vi "PopulateAscriptTree.vi"(10 "Steps in":T1(array[cluster]), 11 "Autoscript Layout":refnum<vi>) -> (0 "error out":errorcluster, 3 "Autoscript Layout":refnum<vi>)   [LabVIEW 2015]
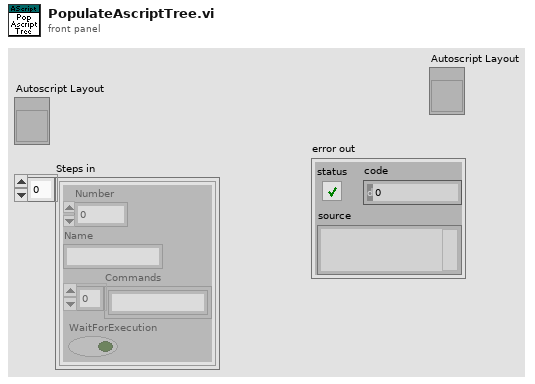
[diagram p1: front panel]
types:
  T1 = cluster{"Number":i32, "Name":string, "Commands":string[], "WaitForExecution":bool}[]
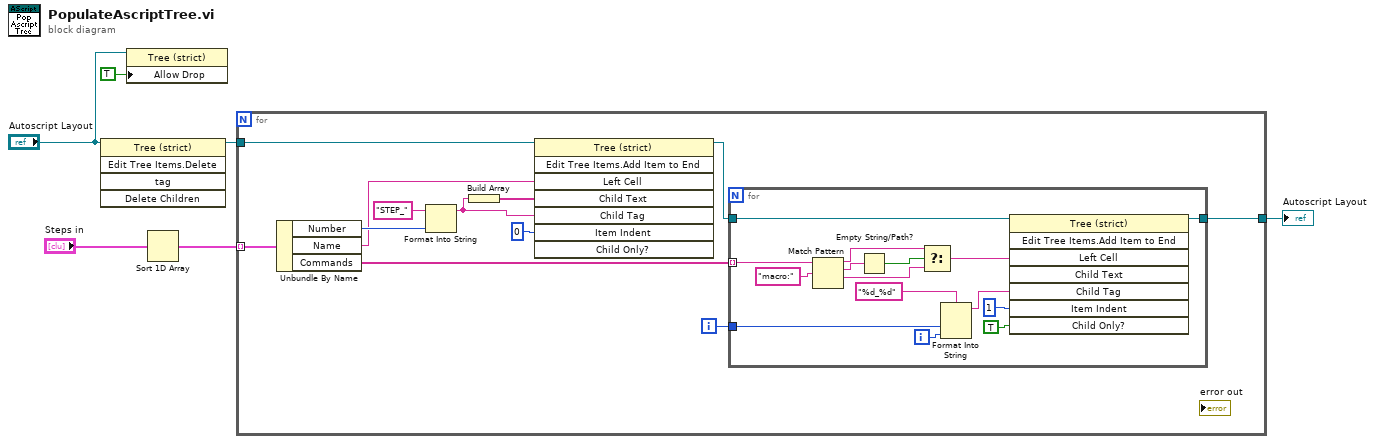
[diagram p0: block diagram]
diagram:
  n1 = invoke class="Tree (strict)" method="Edit Tree Items.Delete"(reference="Autoscript Layout") -> (reference out=w4:refnum<vi>)  [unwired: 4 in, 4 out]
  n2 = property class="Tree (strict)"(reference="Autoscript Layout", "Allow Drop"=TRUE ("Drag/Drop:Allow Dropping")) -> ()  [unwired: 1 in, 2 out]
  n3 = Sort 1D Array(array="Steps in") -> (sorted array=w6:T1)
  n4 = for {
    tunnel: w6 -> [w18] mode=indexing
    tunnel: w4 -> [w17]
    tunnel: [w7] -> w1
    i -> [w8]
    n5 = Unbundle By Name(w18) -> ("Number"=w15:i32, "Name"=w12:string, "Commands"=w11:string[])
    n6 = Format Into String(initial string="STEP_", w15) -> (resulting string=w9:string)  [unwired: 2 in, 1 out]
    n7 = Build Array(w9) -> (w13:string[])
    n8 = invoke class="Tree (strict)" method="Edit Tree Items.Add Item to End"(reference=w17, "Left Cell"=w12, "Child Text"=w13, "Child Tag"=w9, "Item Indent"=0 ("New Item Indentation")) -> (reference out=w10:refnum<vi>)  [unwired: 3 in, 7 out]
    n9 = for {
      tunnel: w10 -> [w33]
      tunnel: w11 -> [w26] mode=indexing
      tunnel: w8 -> [w30]
      tunnel: [w19] -> w7
      i -> [w29]
      n10 = Match Pattern(string=w26, regular expression="macro:") -> (before substring=w22:string, match substring=w24:string, after substring=w21:string)  [unwired: 1 in, 1 out]
      n11 = Empty String/Path?(string/path=w24) -> (empty?=w23:bool)
      n12 = Select(t=w22, s=w23, f=w21) -> (s? t:f=w20:string)
      n13 = Format Into String(format string="%d_%d", w30, w29) -> (resulting string=w28:string)  [unwired: 2 in, 1 out]
      n14 = invoke class="Tree (strict)" method="Edit Tree Items.Add Item to End"(reference=w33, "Left Cell"=w20, "Child Tag"=w28, "Item Indent"=1 ("New Item Indentation"), "Child Only?"=TRUE) -> (reference out=w19:refnum<vi>)  [unwired: 3 in, 7 out]
    }
  }
  "Autoscript Layout" <- w1
